vi "StringIPtoAddress_Simulation.vi"(7 "string IP":string) -> (8 "address":u32)   [LabVIEW 2017]
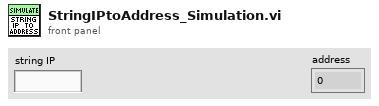
[diagram p1: front panel]
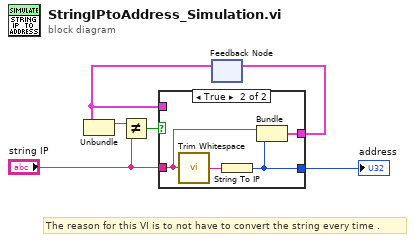
[diagram p0: block diagram]
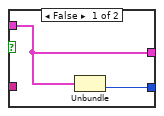
[diagram p2: hidden frame]
diagram:
  # "The reason for this VI is to not have to convert the string every time ."
  n1 = feedback #1() -> (w5:cluster{"string IP":string, u32})  [unwired: 1 in]
  n2 = Unbundle(w5) -> ("string IP"=w3:string)  [unwired: 1 out]
  n3 = Not Equal?(x=w3, y="string IP") -> (x != y?=w2:bool)
  n4 = case shown="True" w2 {
    tunnel: "string IP" -> [_ w11]
    tunnel: [w8 w10] -> w1
    tunnel: w5 -> [w8 _]
    tunnel: [w7 w9] -> w6
    frame False {
      n5 = Unbundle(w8) -> (w7:u32)  [unwired: 1 out]
    }
    frame True {
      n6 = call <vilib>:"Trim Whitespace.vi"("string"=w11) -> ("trimmed string"=w12:string)  [unwired: 1 in]
      n7 = String To IP(1:w12) -> (0:w9:u32)
      n8 = Bundle("string IP"=w11, w9) -> (w10:cluster{"string IP":string, u32})  [unwired: 1 out]
    }
  }
  "address" <- w6
  n9 = feedback-in #1(w1) -> ()
